vi "getSubData_Device_MAGSpec_AllinOne.vi"(9 "variant in":variant, 10 "SubscriberCluster":T1, 11 "timeout":i32=3000) -> (1 "variant out":variant, 2 "OK":bool[](array[boolean]))   [LabVIEW 2013]
uses:
  shared/SubscriberCluster_TypDEf.ctl
  Interface/Sandbox/GUI_Template/GUI_master/tcp_new_data_event.ctl
  Interface/Sandbox/GUI_Template/GUI_master/tcp new data cluster.ctl
  <userlib>/_OpenG.lib/array/array.llb/Remove Duplicates from 1D Array (String)__ogtk.vi
panel:
  out "Data in":string[][](array[string])
  out "time":u32
  out "post time":u32
  out "Waveform Graph":i32[](graph)
  out "Devices 2":string[](array[string])
  out "timed out?":bool
  out "Devices ALL":string[](array[string])
  out "element":string[][](array[string])
  out "Numeric":i32
  out "all lower case string":string[](array[string])
  out "timeout":bool
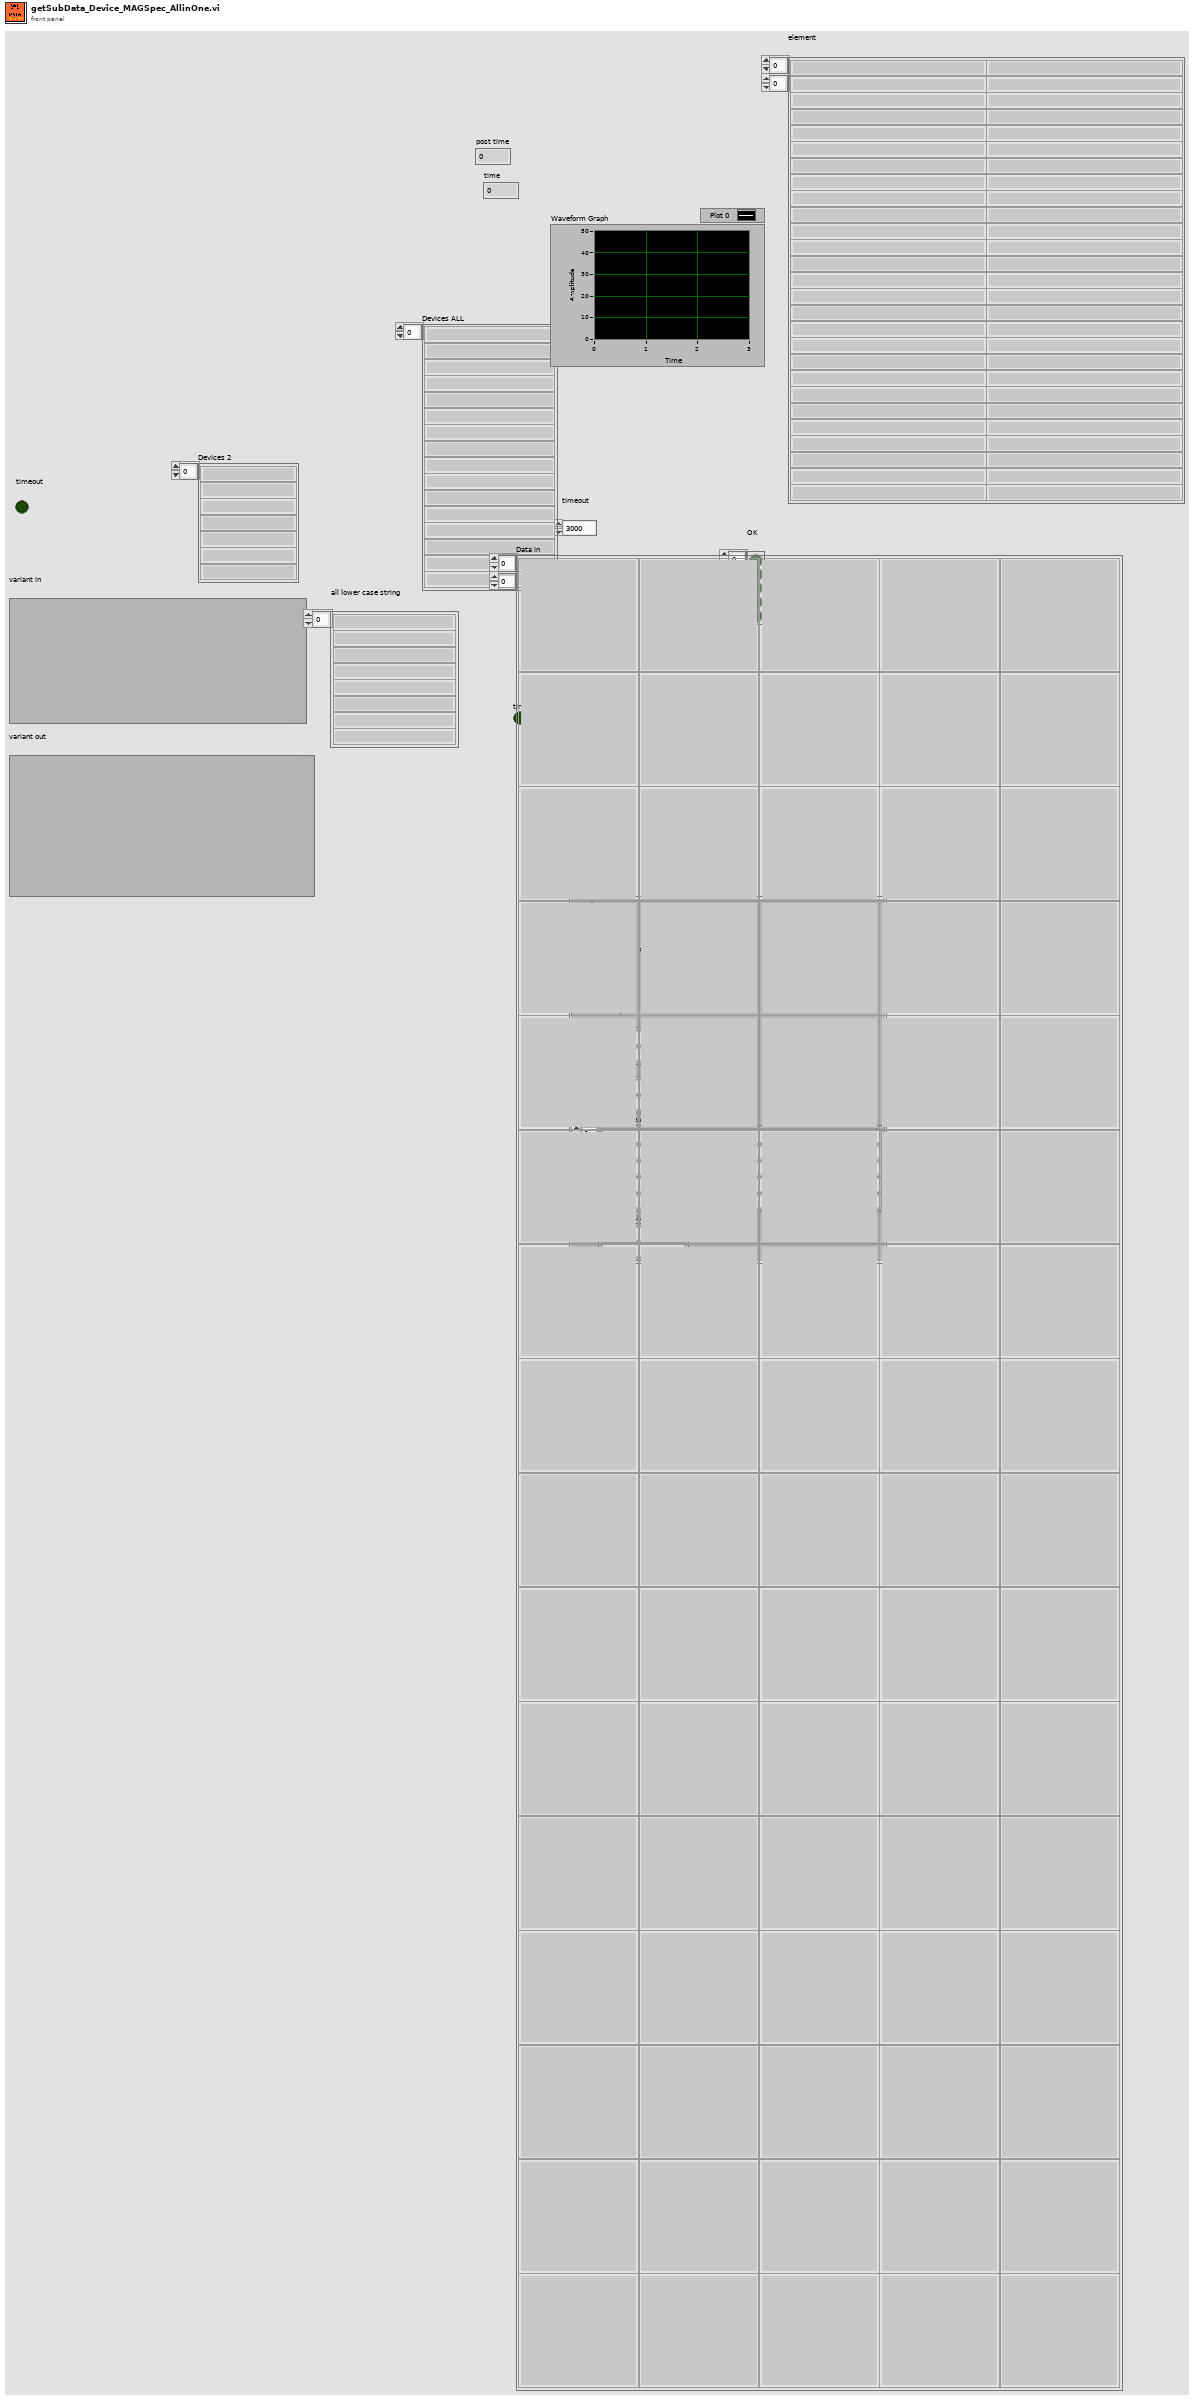
[diagram p1: front panel]
types:
  T1 = typedef "SubscriberCluster_TypDEf.ctl" = cluster{"tcp data event":T2, "Event Registration Refnum":refnum<event-registration>, "data queue":refnum<queue>, "Devices":string[], "Alias":string[], "Variable header":string[], "Devices ALL":string[]}
  T2 = typedef "tcp_new_data_event.ctl" = refnum<user-event>
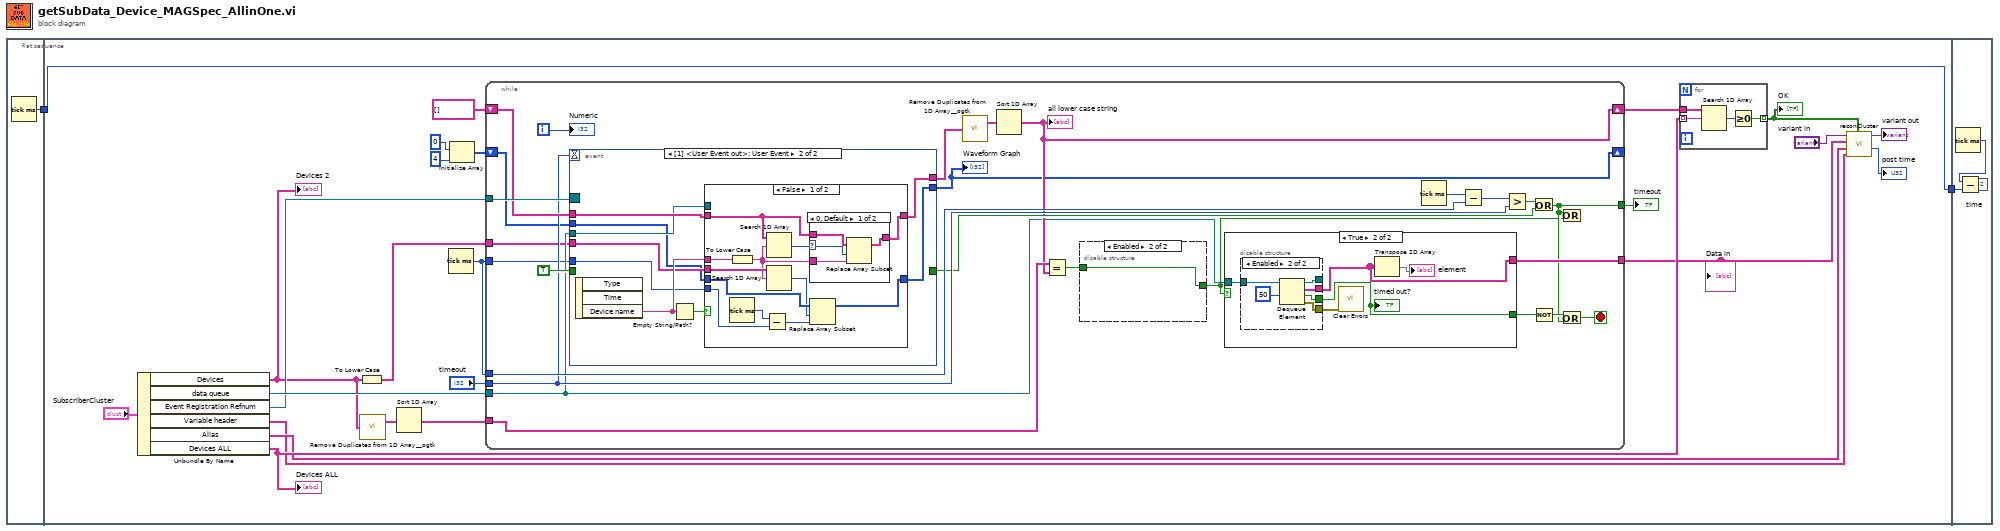
[diagram p0: block diagram]
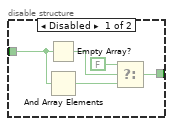
[diagram p2: hidden frame]
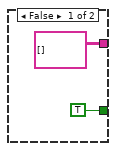
[diagram p3: hidden frame]
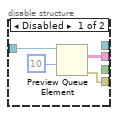
[diagram p4: hidden frame]
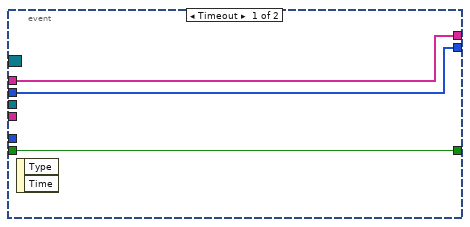
[diagram p5: hidden frame]
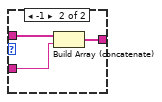
[diagram p6: hidden frame]
diagram:
  n1 = flat-sequence {
    tunnel: [w3] -> w2
    tunnel: w2 -> [w4]
    tunnel: [w4] -> w1
    tunnel: w1 -> [w116]
    frame #0 {
      n2 = Tick Count (ms)() -> (millisecond timer value=w3:u32)
    }
    frame #1 {
      n3 = Unbundle By Name("SubscriberCluster") -> ("Devices"=w17:string[], "data queue"=w24:refnum<queue>, "Event Registration Refnum"=w23:refnum<event-registration>, "Variable header"=w8:string[], "Alias"=w9:string[], "Devices ALL"=w20:string[])
      "Devices ALL" <- w20
      "Devices 2" <- w17
      n4 = To Lower Case(string=w17) -> (all lower case string=w16:string[])
      n5 = call-poly <userlib>:"Remove Duplicates from 1D Array__ogtk.vi"("Input Array"=w17) -> ("Output Array"=w18:string[])  [unwired: 1 out]
      n6 = Sort 1D Array(array=w18) -> (sorted array=w19:string[])
      n7 = Tick Count (ms)() -> (millisecond timer value=w15:u32)
      n8 = Initialize Array(0 ("dimension size"), 4 ("dimension size")) -> (w12:i32[])
      n9 = while {
        tunnel: w23 -> [w57]
        tunnel: w24 -> [w37]
        tunnel: [w47] -> w10
        shift-right: [w44] -> w21
        shift-left: string[] [] -> [w55]
        tunnel: w19 -> [w54]
        tunnel: "timeout" -> [w51]
        tunnel: [w39] -> w22
        tunnel: w15 -> [w53]
        tunnel: w16 -> [w35]
        tunnel: w15 -> [w34]
        shift-right: [w32] -> _
        shift-left: w12 -> [w33]
        i -> [w46]
        stop <- w38 stop-if-true
        n10 = event shown="[1] <User Event out>: User Event" {
          selector: w57 -> [_ _]
          dyn-events: _ -> [_ _]
          timeout: w51 -> [_ _]
          tunnel: [w83 _] -> w50
          tunnel: TRUE -> [w83 _]
          tunnel: [w82 w92] -> w43
          tunnel: w55 -> [w82 w89]
          tunnel: w37 -> [_ w88]
          tunnel: w35 -> [_ w87]
          tunnel: w34 -> [_ w86]
          tunnel: w33 -> [w81 w85]
          tunnel: [w81 w84] -> w32
          event Timeout {
            n11 = event-data() -> ()  [unwired: 1 in, 2 out]
          }
          event User Event {
            n12 = event-data() -> ("Device name"=w91:string)  [unwired: 1 in, 2 out]
            n13 = Empty String/Path?(string/path=w91) -> (empty?=w90:bool)
            n14 = case shown="False" w90 {
              tunnel: w91 -> [w101 _]
              tunnel: [w104 w113] -> w92
              tunnel: w89 -> [w103 w113]
              tunnel: w88 -> [_ _]
              tunnel: w87 -> [w100 _]
              tunnel: w86 -> [w97 _]
              tunnel: w85 -> [w96 w112]
              tunnel: [w93 w112] -> w84
              frame False {
                n15 = To Lower Case(string=w101) -> (all lower case string=w99:string)
                n16 = Tick Count (ms)() -> (millisecond timer value=w98:u32)
                n17 = Subtract(x=w98, y=w97) -> (x-y=w95:u32)
                n18 = Search 1D Array(1D array=w103, element=w99) -> (index of element=w102:i32)  [unwired: 1 in]
                n19 = Search 1D Array(1D array=w100, element=w99) -> (index of element=w94:i32)  [unwired: 1 in]
                n20 = case shown="0, Default" w102 {
                  selector: w102 -> [w106 _]
                  tunnel: w99 -> [w105 w111]
                  tunnel: [w107 w110] -> w104
                  tunnel: w103 -> [w108 w109]
                  frame 0, Default {
                    n21 = Replace Array Subset(array=w108, new element=w105, index=w106) -> (w107:string[])
                  }
                  frame -1 {
                    n22 = Build Array (concatenate)(w109, w111) -> (w110:string[])
                  }
                }
                n23 = Replace Array Subset(array=w96, new element=w95, index=w94) -> (w93:i32[])
              }
              frame True {
              }
            }
          }
        }
        "Waveform Graph" <- w32
        n24 = call-poly <userlib>:"Remove Duplicates from 1D Array__ogtk.vi"("Input Array"=w43) -> ("Output Array"=w42:string[])  [unwired: 1 out]
        n25 = Sort 1D Array(array=w42) -> (sorted array=w44:string[])
        "all lower case string" <- w44
        n26 = Equal?(x=w54, y=w44) -> (x = y?=w45:bool)
        n27 = disable-structure shown="Enabled" {
          disable-tunnel: w45 -> [w62 w63]
          disable-tunnel: [w58 w63] -> w36
          frame Disabled {
            n28 = Empty Array?(array=w62) -> (empty?=w61:bool)
            n29 = And Array Elements(Boolean array=w62) -> (logical AND=w59:bool)
            n30 = Select(t=FALSE ("empty?"), s=w61, f=w59) -> (s? t:f=w58:bool)
          }
          frame Enabled {
          }
        }
        n31 = case shown="True" w36 {
          tunnel: w37 -> [_ w70]
          tunnel: [string[][] [] ("Data in") w67] -> w47
          tunnel: [TRUE ("timed out?") w68] -> w41
          frame False {
          }
          frame True {
            n32 = disable-structure shown="Enabled" {
              disable-tunnel: w70 -> [w73 w80]
              disable-tunnel: [w72 w79] -> w67
              disable-tunnel: [w71 w78] -> w69
              disable-tunnel: [_ w76] -> _
              disable-tunnel: [_ w75] -> w68
              frame Disabled {
                n33 = Preview Queue Element(queue=w73, timeout in ms (-1)=10) -> (element=w72:string[][], error out=w71:errorcluster)  [unwired: 1 in, 2 out]
              }
              frame Enabled {
                n34 = Dequeue Element(queue=w80, timeout in ms (-1)=50) -> (queue out=w76:refnum<queue>, element=w79:string[][], timed out?=w75:bool, error out=w78:errorcluster)  [unwired: 1 in]
              }
            }
            "timed out?" <- w68
            n35 = call <vilib>:"Clear Errors.vi"("error in (no error)"=w69) -> ()  [unwired: 6 in, 1 out]
            n36 = Transpose 2D Array(2D array=w67) -> (transposed array=→"element":string[][])
          }
        }
        n37 = Tick Count (ms)() -> (millisecond timer value=w48:u32)
        n38 = Subtract(x=w48, y=w53) -> (x-y=w52:u32)
        n39 = Greater?(x=w52, y=w51) -> (0:w49:bool)
        n40 = Or(x=w49, y=w50) -> (x .or. y?=w39:bool)
        n41 = Not(x=w41) -> (.not. x?=w40:bool)
        n42 = Or(x=w39, y=w36) -> ()  [unwired: 1 out]
        n43 = Or(x=w40, y=w39) -> (x .or. y?=w38:bool)
        "Numeric" <- w46
      }
      "timeout" <- w22
      "Data in" <- w10
      n44 = for {
        tunnel: w20 -> [w30] mode=indexing
        tunnel: w21 -> [w31]
        tunnel: [w28] -> w6 mode=indexing
        n45 = Search 1D Array(1D array=w31, element=w30) -> (index of element=w29:i32)  [unwired: 1 in]
        n46 = Greater Or Equal To 0?(x=w29) -> (x >= 0?=w28:bool)
      }
      "OK" <- w6
      n47 = call "reconCluster.vi"("Array 6"=w6, "Variable header"=w8, "Alias"=w9, "Data in"=w10, "variant in"="variant in") -> ("time"=→"post time":u32, "variant out"=→"variant out":variant)  [unwired: 5 in]
    }
    frame #2 {
      n48 = Tick Count (ms)() -> (millisecond timer value=w115:u32)
      n49 = Subtract(x=w115, y=w116) -> (x-y=→"time":u32)
    }
  }
